vi "Dateischreiben_Einkanal_V3Hadware .vi"() -> ()   [LabVIEW 2016]
uses:
  <vilib>/express/express shared/transition.llb/Dynamic To Waveform Array.vi
  <vilib>/express/express arith-compare/Formula/Block/exnFormulaBlock how many pts in the wave.vi
  <vilib>/express/express shared/ex_Modify Signal Name.vi
  <vilib>/express/express shared/transition.llb/Waveform Array To Dynamic.vi
  <vilib>/express/express arith-compare/Formula/XNode/ExpressFormulaBlockNode.xnode
panel:
  out "Volumen":dynamicdata(graph)
  out "TE_U":dbl
  out "PT_U":dbl
  in  "Messfrequenz":dbl=10.0
  in  "Spalten":string[](array[string])=["t(s)\n", "PT_U", "TE_U", "PT_T", "TE_T"]
  in  "Header":string[](array[string])=["Messlabor\n", "sr", "Alex Uhl", "HTBLA Kaindorf"]
  out "Volumensstrom":dynamicdata(graph)
  in  "Eingangs-String":string="%f\\t%f\\t%f\\t%f\\t%f\\n"
  in  "Pfad":path=path "C:/Users/Messlabor_Kustos/Desktop/Schueler/4BHME/UhlTrauß_Einheit4/einheit4.xls"
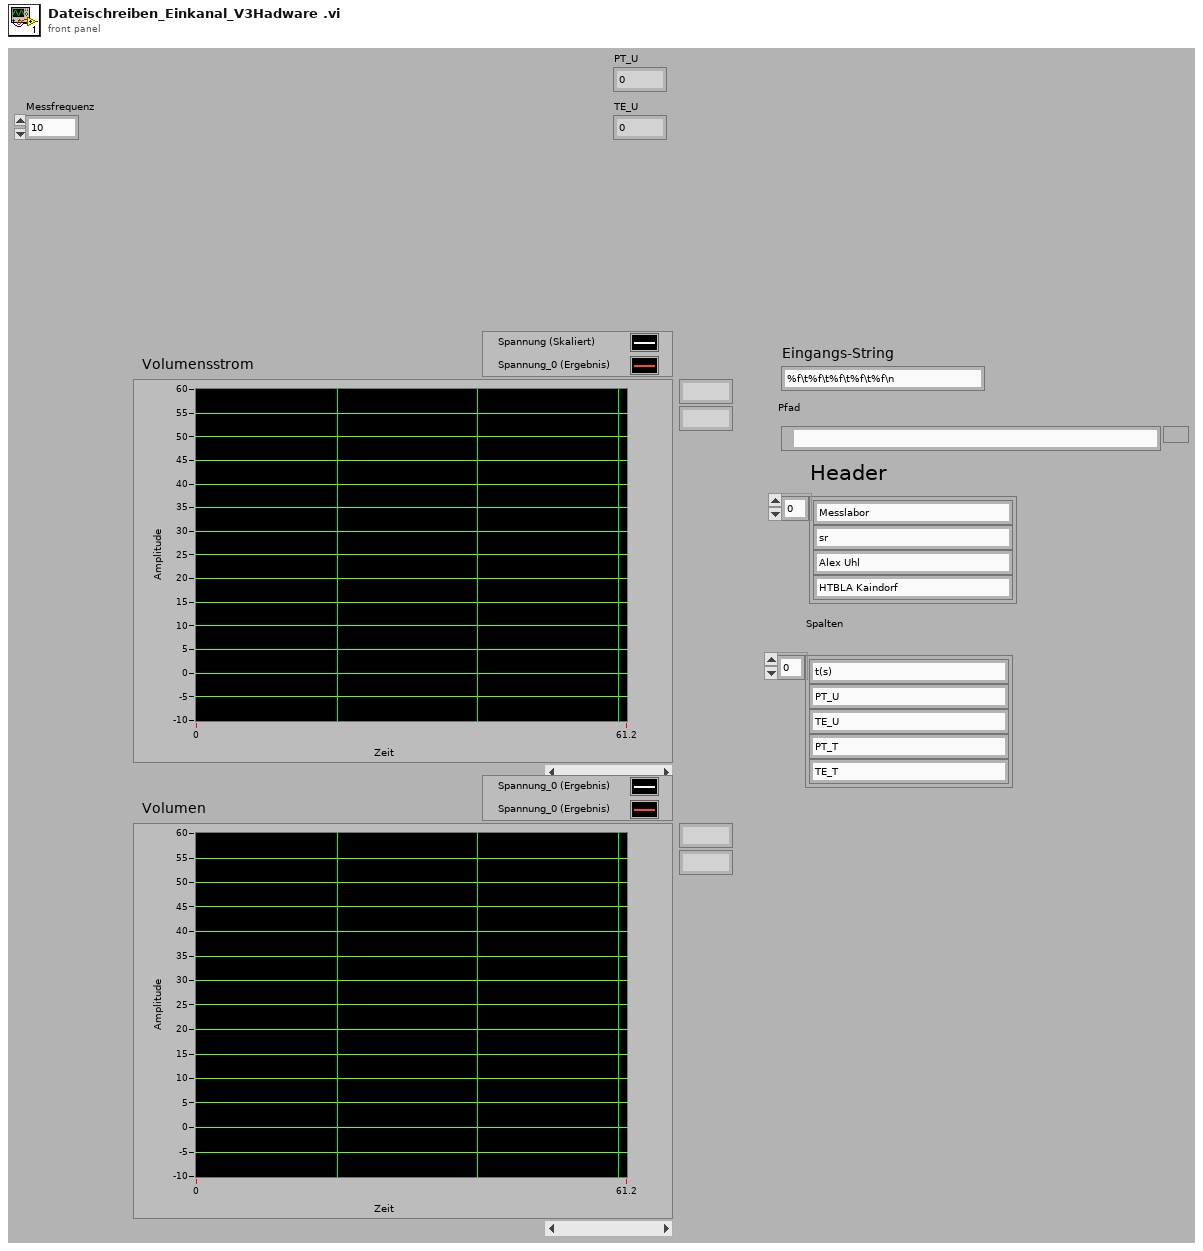
[diagram p1: front panel]
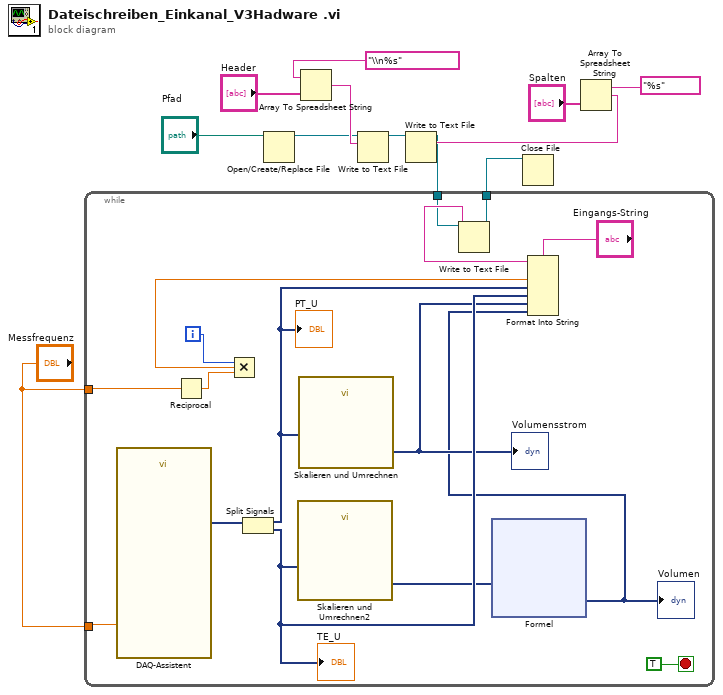
[diagram p0: block diagram]
diagram:
  n1 = Open/Create/Replace File(file path (use dialog)="Pfad") -> (refnum out=w1:refnum<file>)  [unwired: 5 in, 2 out]
  n2 = Array To Spreadsheet String(array="Header", 3:"\\n%s" ("Format-String")) -> (spreadsheet string=w6:string)  [unwired: 1 in]
  n3 = Write to Text File(file (use dialog)=w1, text=w6) -> (refnum out=w3:refnum<file>)  [unwired: 2 in, 2 out]
  n4 = Array To Spreadsheet String(array="Spalten", 3:"%s" ("Format-String")) -> (spreadsheet string=w5:string)  [unwired: 1 in]
  n5 = Write to Text File(file (use dialog)=w3, text=w5) -> (refnum out=w4:refnum<file>)  [unwired: 2 in, 2 out]
  n6 = while {
    tunnel: [w28] -> w12
    tunnel: w4 -> [w24]
    tunnel: "Messfrequenz" -> [w20]
    tunnel: "Messfrequenz" -> [w16]
    i -> [w22]
    stop <- TRUE stop-if-true
    n7 = call "DAQ-Assistent"("Rate"=w16) -> ("data"=w17:dynamicdata)  [unwired: 15 in, 3 out]
    n8 = Reciprocal(x=w20) -> (1/x=w23:dbl)
    n9 = Multiply(x=w22, y=w23) -> (x*y=w21:dbl)
    n10 = Split Signals(w17) -> (w19:dynamicdata, w18:dynamicdata)  [unwired: 2 in]
    "PT_U" <- w19
    "TE_U" <- w18
    n11 = call "Skalieren und Umrechnen2"("Signals"=w18) -> ("Scaled Signals"=w15:dynamicdata)  [unwired: 9 in, 1 out]
    n12 = call "Skalieren und Umrechnen"("Signals"=w19) -> ("Scaled Signals"=w14:dynamicdata)  [unwired: 9 in, 1 out]
    "Volumensstrom" <- w14
    n13 = xnode "Formel"("X1"=w15) -> ("Ergebnis"=w13:dynamicdata)  [unwired: 1 in, 1 out]
    "Volumen" <- w13
    n14 = Format Into String(format string="Eingangs-String", w21, w19, w18, w14, w13) -> (resulting string=w27:string)  [unwired: 2 in, 1 out]
    n15 = Write to Text File(file (use dialog)=w24, text=w27) -> (refnum out=w28:refnum<file>)  [unwired: 2 in, 2 out]
  }
  n16 = Close File(refnum=w12) -> ()  [unwired: 1 in, 2 out]
